vi "Initialize Arduino.vi"(8 "error in (no error)":errorcluster, 11 "VISA Refnum in":refnum<visa-resource-name>) -> (0 "error out":errorcluster, 3 "COM port out":refnum<visa-resource-name>)   [LabVIEW 2020]
uses:
  Controls/LED panel ---typedef.ctl
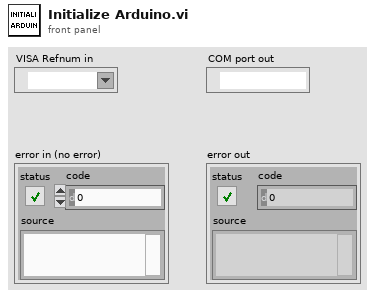
[diagram p1: front panel]
types:
  T1 = typedef "LED panel ---typedef.ctl" = cluster{"R":bool, "G":bool, "B":bool, "W":bool}
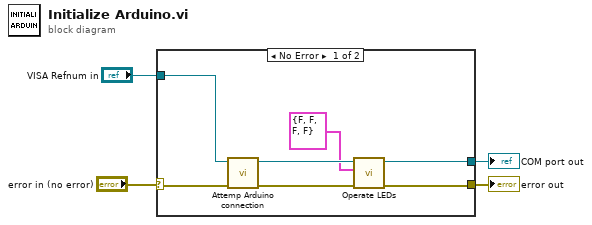
[diagram p0: block diagram]
diagram:
  n1 = case shown="No Error" "error in (no error)" {
    selector: "error in (no error)" -> [w8 w13]
    tunnel: [w10 w13] -> w4
    tunnel: "VISA Refnum in" -> [w7 w12]
    tunnel: [w5 w12] -> w1
    frame No Error {
      n2 = call "Attemp Arduino connection.vi"("error in (no error)"=w8, "COM port in"=w7) -> ("error out"=w9:errorcluster, "COM port out"=w11:refnum<visa-resource-name>)  [unwired: 8 in]
      n3 = call "Operate LEDs.vi"("error in (no error)"=w9, "LED Panel"=T1 {"R"=FALSE, "G"=FALSE, "B"=FALSE, "W"=FALSE}, "COM port in"=w11) -> ("error out"=w10:errorcluster, "COM port out"=w5:refnum<visa-resource-name>)  [unwired: 7 in]
    }
    frame Error {
    }
  }
  "error out" <- w4
  "COM port out" <- w1
